vi "Write Support Runtime Configuration.vi"(8 "error in":errorcluster, 10 "Support Runtime Configuration":bool, 11 "NIVS_CD Template in":refnum<class "NIVS_CD Template.lvclass">) -> (0 "error out":errorcluster, 3 "NIVS_CD Template out":refnum<class "NIVS_CD Template.lvclass">)   [LabVIEW 2020, in "NIVS_CD Template.lvclass"]
uses:
  NIVS_CD Template.lvclass
  NIVS_CD Template.lvclass/NIVS_CD Template.ctl
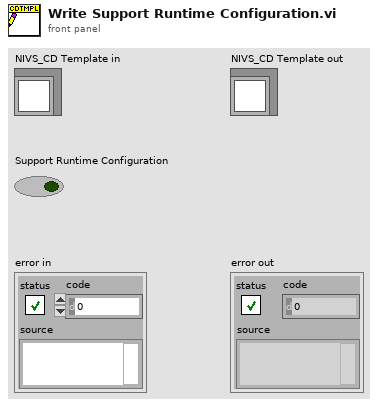
[diagram p1: front panel]
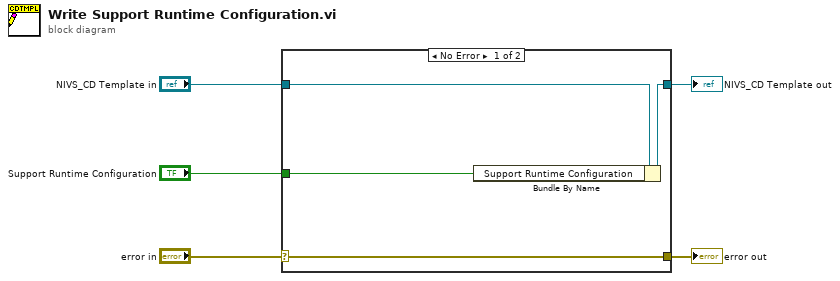
[diagram p0: block diagram]
diagram:
  n1 = case shown="No Error" "error in" {
    selector: "error in" -> [w9 w11]
    tunnel: [w9 w11] -> w4
    tunnel: [w7 w10] -> w2
    tunnel: "NIVS_CD Template in" -> [w8 w10]
    tunnel: "Support Runtime Configuration" -> [w6 _]
    frame No Error {
      n2 = Bundle By Name(cluster=w8, "Support Runtime Configuration"=w6) -> (w7:refnum<class "NIVS_CD Template.lvclass">)
    }
    frame Error {
    }
  }
  "error out" <- w4
  "NIVS_CD Template out" <- w2
